vi "sedSpectrometer_putSample_SpectTemperature.vi"(8 "error in (no error)":errorcluster, 11 "SpectTemperature_Ctl":T1) -> (0 "error out":errorcluster, 2 "function return":i32, 3 "SpectTemperature_Ctl out":T1)   [LabVIEW 2016, in "SALLV_sedSpectrometer.lvlib"]
doc: "int sedSpectrometer_shm_putSample_SpectTemperatureLV(sedSpectrometer_SpectTemperatureLV *SpectTemperature_Ctl );"
uses:
  SALLV_sedSpectrometer.lvlib
  DataTypes/SpectTemperature.ctl
  SALLV_sedSpectrometer.so
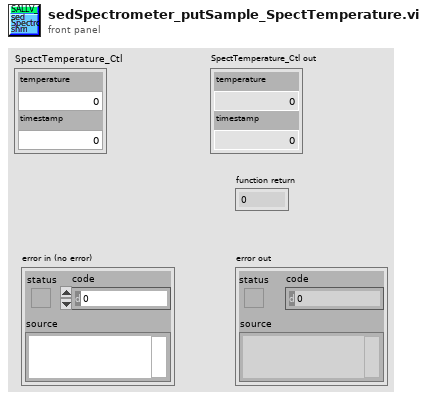
[diagram p1: front panel]
types:
  T1 = typedef "SALLV_sedSpectrometer.lvlib/SpectTemperature.ctl" = cluster{"temperature":dbl, "timestamp":dbl}
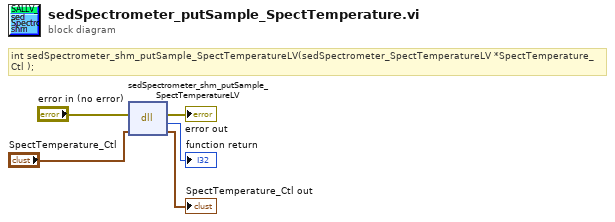
[diagram p0: block diagram]
diagram:
  # "int sedSpectrometer_shm_putSample_SpectTemperatureLV(sedSpectrometer_SpectTemperatureLV *SpectTemperature_Ctl );"
  n1 = dll-call lib="home/harini/TCS/ts_sallv_sedSpectrometer_371/SALLV_sedSpectrometer.*" fn="sedSpectrometer_shm_putSample_SpectTemperatureLV"(error in="error in (no error)", "SpectTemperature_Ctl"="SpectTemperature_Ctl") -> (error out=→"error out":errorcluster, →"function return":i32, "SpectTemperature_Ctl"=→"SpectTemperature_Ctl out":T1)  [unwired: 2 in, 1 out]
